vi "DB Tools Insert Data EDITED.vi"(8 "error_in":errorcluster, 10 "INSERT_statement":string, 11 "connection_reference_in":T1) -> (0 "error_out":errorcluster, 1 "SQL_result":variant[][](array[variant]), 3 "connection_reference_out":T1, 4 "executed_SQL_statement":string)   [LabVIEW 2020]
doc: "This is edited version of DB Tools Select Data vi from NI Database Connectivity Toolkit, with added functionality to limit number of row selected. Also added output with exact SQL statement sent to database. PROCEED WITH CARE (JL)"
uses:
  <vilib>/addons/database/Connection.llb/Conn ObjectReference.ctl
  SQL_statement_type.ctl
  <vilib>/addons/database/Connection.llb/Conn Execute.vi
  <vilib>/addons/database/Recordset.llb/Rec Fetch Recordset Data (R).vi
  <vilib>/addons/database/Recordset.llb/Rec Destroy - Connection.vi
  <vilib>/addons/database/NI_Database_API.lvlib
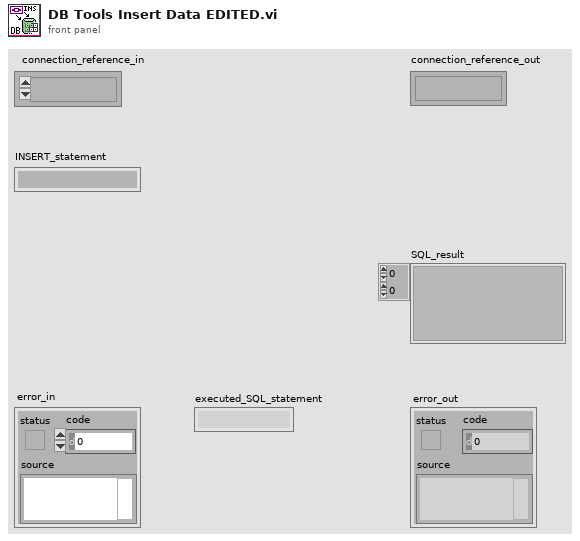
[diagram p1: front panel]
types:
  T1 = typedef "NI_Database_API.lvlib/Conn ObjectReference.ctl" = refnum<k1>
  T2 = typedef "SQL_statement_type.ctl" = enum16{"SELECT", "INSERT", "UPDATE", "DELETE"}
  T3 = typedef "NI_Database_API.lvlib/Rec ObjectReference.ctl" = refnum<k1>
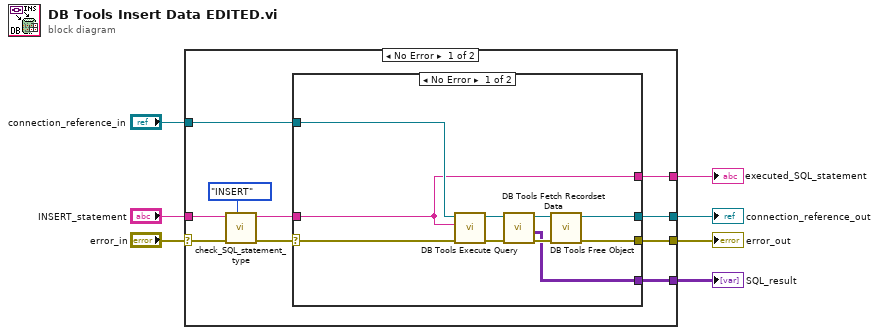
[diagram p0: block diagram]
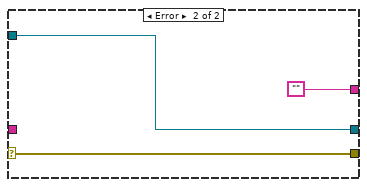
[diagram p2: hidden frame]
diagram:
  n1 = case shown="No Error" "error_in" {
    selector: "error_in" -> [w10 w33]
    tunnel: "INSERT_statement" -> [w13 _]
    tunnel: [w17 w33] -> w6
    tunnel: [w16 w32] -> w5
    tunnel: "connection_reference_in" -> [w15 w32]
    tunnel: [w14 ""] -> w2
    tunnel: [w8 _] -> w1
    frame No Error {
      n2 = call "check_SQL_statement_type.vi"("SQL_statement_type"=SQL_statement_type."INSERT", "error_in"=w10, "SQL_statement_in"=w13) -> ("error_out"=w9:errorcluster, "SQL_statement_out"=w12:string)  [unwired: 7 in]
      n3 = case shown="No Error" w9 {
        selector: w9 -> [w24 w30]
        tunnel: [w25 w30] -> w17
        tunnel: [w27 w29] -> w16
        tunnel: w15 -> [w26 w29]
        tunnel: [w23 ""] -> w14
        tunnel: w12 -> [w23 _]
        tunnel: [w18 _] -> w8
        frame No Error {
          n4 = call-poly <vilib>:"DB Tools Execute Query.vi"("error in (no error)"=w24, "SQL query"=w23, "connection reference"=w26) -> ("error out"=w20:errorcluster, "recordset reference"=w22:T3)  [unwired: 5 in]
          n5 = call-poly <vilib>:"DB Tools Fetch Recordset Data.vi"("error in (no error)"=w20, "recordset reference"=w22) -> ("error out"=w19:errorcluster, "recordset data"=w18:variant[][], "recordset reference out"=w21:T3)  [unwired: 3 in]
          n6 = call-poly <vilib>:"DB Tools Free Object.vi"("error in (no error)"=w19, "recordset reference"=w21) -> ("error out"=w25:errorcluster, "connection reference"=w27:T1)  [unwired: 8 in]
        }
        frame Error {
        }
      }
    }
    frame Error {
    }
  }
  "error_out" <- w6
  "connection_reference_out" <- w5
  "executed_SQL_statement" <- w2
  "SQL_result" <- w1
